vi "LoadState.vi"(8 "error in (no error)":errorcluster, 10 "Load":bool, 11 "VISA Refnum in":refnum<visa-resource-name>) -> (0 "error out":errorcluster, 3 "VISA Refnum out":refnum<visa-resource-name>)   [LabVIEW 2020]
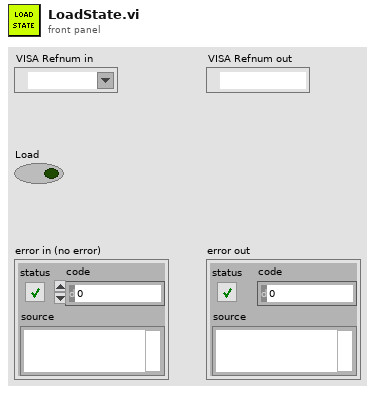
[diagram p1: front panel]
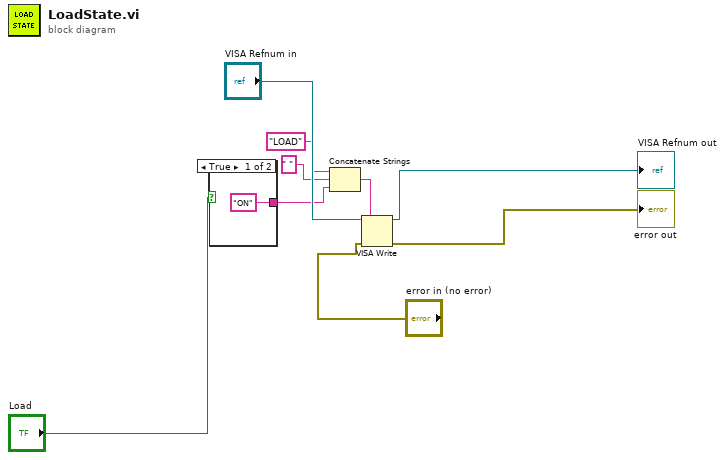
[diagram p0: block diagram]
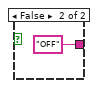
[diagram p2: hidden frame]
diagram:
  n1 = case shown="True" "Load" {
    tunnel: ["ON" ("string") "OFF" ("string")] -> w4
    frame True {
    }
    frame False {
    }
  }
  n2 = Concatenate Strings("LOAD" ("string"), " " ("string"), w4) -> (w5:string)
  n3 = VISA Write(VISA resource name="VISA Refnum in", write buffer=w5, error in (no error)="error in (no error)") -> (VISA resource name out=→"VISA Refnum out":refnum<visa-resource-name>, error out=→"error out":errorcluster)  [unwired: 1 out]
